vi "FTW-Container-Value-Enum.vi"(0 "JSON":refnum<class "FTW-Container.lvclass">, 11 "error in":errorcluster) -> (4 "JSON out":refnum<class "FTW-Container.lvclass">, 6 "Value":u64, 8 "String":string, 15 "error out":errorcluster)   [LabVIEW 2015, in "FTW-Container.lvclass"]
uses:
  FTW-Container.lvclass
  FTW-Container.lvclass/FTW-Container.ctl
  <vilib>/Utility/Data Type/NI_Data Type.lvlib
panel:
  # "Inputs"
  # "Outputs"
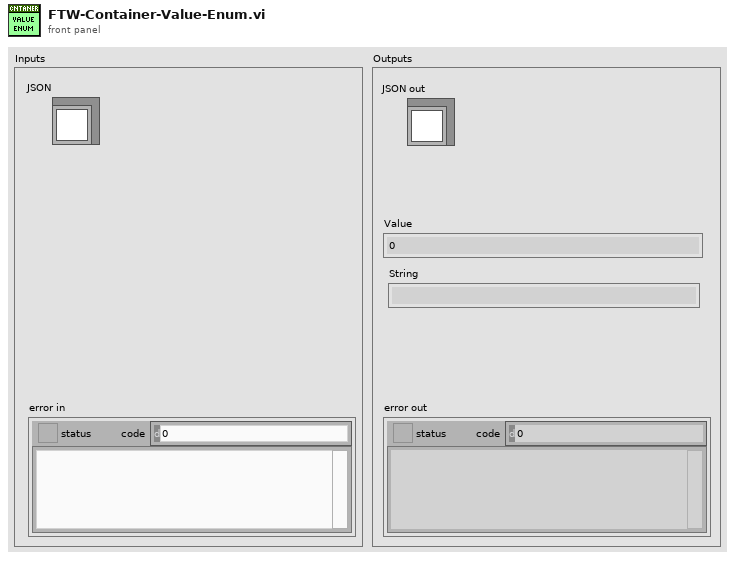
[diagram p1: front panel]
types:
  T1 = typedef "NI_Data Type.lvlib/Data Type.ctl" = enum8{"Invalid Type", "Void", "I8", "I16", "I32", "I64", "U8", "U16", "U32", "U64", "Single Float", "Double Float", "Extended Float", "Single Complex", "Double Complex", "Extended Complex", "Enum U8", "Enum U16", "Enum U32", "Enum U64", "Single Float With Unit", "Double Float With Unit", "Extended Float With Unit", "Single Complex with Unit", "Double Complex with Unit", "Extended Complex with Unit", "Boolean", "String", "Path", "Picture", "Tag", "Array", "Cluster", "Variant", "LV Variant", "Waveform", "Timestamp", "Digital Waveform", "Digital Data", "ExpressData", "Refnum", "External Data", "VI", "Poly VI", "LabVIEW Class Instance", "Fixed Point"}
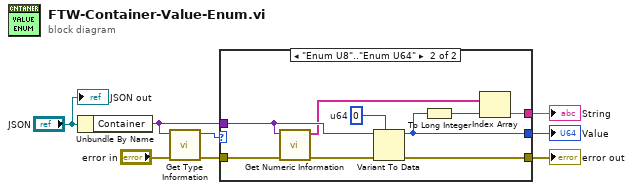
[diagram p0: block diagram]
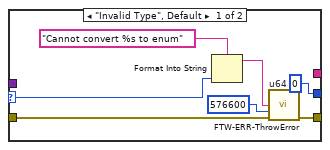
[diagram p2: hidden frame]
diagram:
  n1 = Unbundle By Name("JSON") -> ("Container"=w2:variant)
  n2 = call <vilib>:"Get Type Information.vi"("error in (no error)"="error in", "Variant"=w2) -> ("error out"=w8:errorcluster, "Type"=w7:T1)  [unwired: 5 in, 3 out]
  n3 = case shown="\"Enum U8\"..\"Enum U64\"" w7 {
    selector: w7 -> [w11 _]
    tunnel: w8 -> [w14 w23]
    tunnel: w2 -> [_ w20]
    tunnel: [w13 w22] -> w5
    tunnel: [w15 w19] -> w4
    tunnel: [_ w17] -> w1
    frame "Invalid Type", Default {
      w15 = u64 0  # u64
      n4 = Format Into String(format string="Cannot convert %s to enum" ("Error Message"), w11) -> (resulting string=w9:string)  [unwired: 2 in, 1 out]
      n5 = call "FTW-ERR-ThrowError.vi"("Error Message"=w9, "Error Code"=576600, "error in"=w14) -> ("error out"=w13:errorcluster)  [unwired: 12 in]
    }
    frame "Enum U8".."Enum U64" {
      w24 = u64 0  # u64
      n6 = call <vilib>:"Get Numeric Information.vi"("error in (no error)"=w23, "Variant"=w20) -> ("error out"=w21:errorcluster, "Enum Names"=w18:string[])  [unwired: 6 in, 2 out]
      n7 = Variant To Data(error in=w21, type=w24, Variant=w20) -> (data=w19:u64, error out=w22:errorcluster)
      n8 = To Long Integer(number=w19) -> (32bit integer=w16:i32)
      n9 = Index Array(array=w18, index=w16) -> (element=w17:string)
    }
  }
  "error out" <- w5
  "Value" <- w4
  "String" <- w1
  "JSON out" <- "JSON"
